vi "SetLevel.vi"(8 "error in (no error)":errorcluster, 10 "Level (dBm)":dbl, 11 "NetA_RSZVL in":refnum<class "NetA_RSZVL.lvclass">) -> (0 "error out":errorcluster, 3 "NetA_RSZVL out":refnum<class "NetA_RSZVL.lvclass">)   [LabVIEW 2014, in "NetA_RSZVL.lvclass"]
uses:
  NetA_RSZVL.lvclass
  NetA_RSZVL.lvclass/NetA_RSZVL.ctl
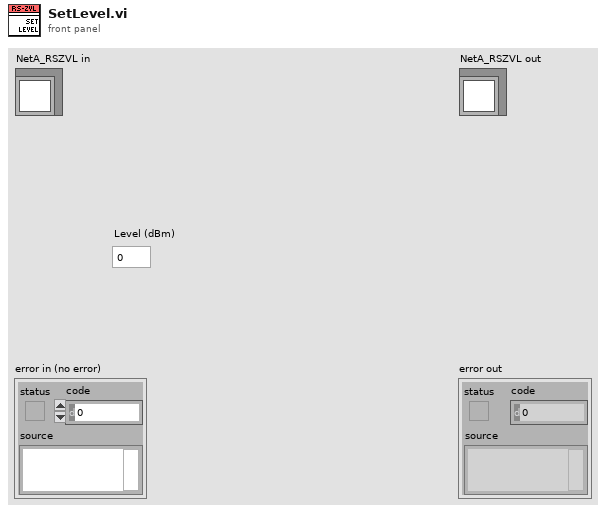
[diagram p1: front panel]
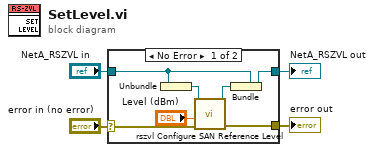
[diagram p0: block diagram]
diagram:
  n1 = case shown="No Error" "error in (no error)" {
    selector: "error in (no error)" -> [w9 w13]
    tunnel: "NetA_RSZVL in" -> [w8 w12]
    tunnel: [w6 w12] -> w2
    tunnel: [w5 w13] -> w1
    frame No Error {
      n2 = Unbundle(w8) -> (w11:refnum<visa-resource-name>)
      n3 = call <instrlib>:"rszvl Configure SAN Reference Level.vi"("error in (no error)"=w9, "Reference Level (-20.0)"="Level (dBm)", "VISA resource name"=w11) -> ("error out"=w5:errorcluster, "VISA resource name out"=w7:refnum<visa-resource-name>)  [unwired: 7 in]
      n4 = Bundle(cluster=w8, w7) -> (w6:refnum<class "NetA_RSZVL.lvclass">)
    }
    frame Error {
    }
  }
  "error out" <- w1
  "NetA_RSZVL out" <- w2
